vi "Measurement.UI.SetControllerDependency.vi"(8 "error in (no error)":errorcluster, 10 "Measurement":refnum<class "Measurement.lvclass">, 11 "Measurement.IVCurve.UI in":refnum<class "Measurement.IVCurve.UI.lvclass">) -> (0 "error out":errorcluster, 3 "Measurement.IVCurve.UI out":refnum<class "Measurement.IVCurve.UI.lvclass">)   [LabVIEW 2017, in "Measurement.IVCurve.UI.lvclass"]
uses:
  Measurement.IVCurve.UI.lvclass
  Measurement/Measurement.lvclass
  Measurement.IVCurve/Measurement.IVCurve.lvclass
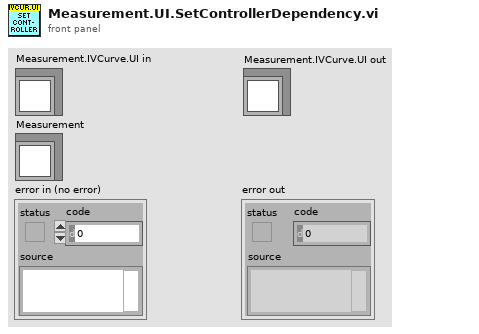
[diagram p1: front panel]
types:
  T1 = typedef "Measurement.IVCurve.UI.lvclass/Dependencies--Cluster.ctl" = cluster{"Measurement.IVCurve":refnum<class "Measurement.IVCurve.lvclass">}
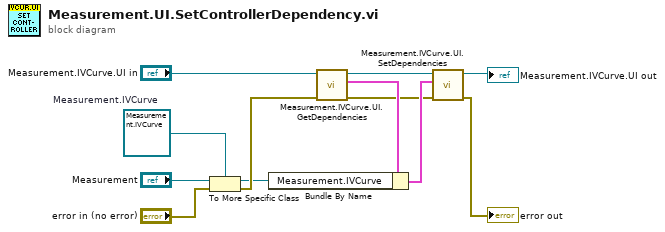
[diagram p0: block diagram]
diagram:
  w1 = refnum<class "Measurement.IVCurve.lvclass"> refnum  # Measurement.IVCurve
  n1 = To More Specific Class(target class=w1, reference="Measurement", error in="error in (no error)") -> (specific class reference=w7:refnum<class "Measurement.IVCurve.lvclass">, error out=w9:errorcluster)
  n2 = call "Measurement.IVCurve.UI.GetDependencies.vi"("error in (no error)"=w9, "Measurement.IVCurve.UI in"="Measurement.IVCurve.UI in") -> ("error out"=w5:errorcluster, "Dependencies"=w8:T1, "Measurement.IVCurve.UI out"=w4:refnum<class "Measurement.IVCurve.UI.lvclass">)  [unwired: 7 in]
  n3 = Bundle By Name(cluster=w8, "Measurement.IVCurve"=w7) -> (w6:T1)
  n4 = call "Measurement.IVCurve.UI.SetDependencies.vi"("error in (no error)"=w5, "Dependencies"=w6, "Measurement.IVCurve.UI in"=w4) -> ("error out"=→"error out":errorcluster, "Measurement.IVCurve.UI out"=→"Measurement.IVCurve.UI out":refnum<class "Measurement.IVCurve.UI.lvclass">)  [unwired: 7 in]
